vi "Mod_OFDM_Set_Ofdm_Frame.vi"(0 "Configure Variant":variant, 7 "ADD Symbol":T2, 9 "Add/delete":bool, 11 "error in":errorcluster, 12 "Edit Position":cluster{"Row":i32, "Column":i32}={"Row"=1000, "Column"=0} {"Row" min=0}) -> (4 "Configure Variant":variant, 8 "OFDM Frame":T1(array[cluster]), 15 "error out":errorcluster)   [LabVIEW 2010]
uses:
  Controls(Type_DEf)/Attribute Data Types.ctl
  Controls(Type_DEf)/Configure Pulse Shaping.ctl
  Controls(Type_DEf)/Pool of Modulator Control.ctl
  Controls(Type_DEf)/Pool of Data Source Control.ctl
  Controls(Type_DEf)/Attribute Names.ctl
  Mod_OFDM_Get_OFDM_Frame.vi
panel:
  in  "Attribute Data Types":T3={"Pulse Shaping"={"System Filter"={"TX Filter"=enum."none", "Alpha"=0.0, "filter length"=0}, "Modulation system parameters"={"samples per symbol (16)"=0}, "symbol rate (Hz)"=0.0}, "FRAME Table"=[], "OFDM Frame"=[], "Sub Carrier Selection"={"Sub Carrier Selection"=[], "OFDM Parameters"={"# of Sub Carrier"=0, "Length Of Cylic Prefix"=0}}, "Symbol Table"=[], "Symbol Pool"=[], "Pool of Modulators"=[], "Pool of Data Sources"=[], "Atribute Names"={"Data Source Pool"="Data Source Pool ", "Modulator Source Pool"="Modulator Source Pool ", "OFDM SYMBOL POOL"="OFDM SYMBOL POOL", "Symbol Table"="Symbol Table", "Sub Carrier Selection"="Sub Carrier Selection", "OFDM Frame"="OFDM Frame", "FRAME Table"="FRAME Table", "Pulse Shaping"="Pulse Shaping"}} {"Pool of Data Sources"."Register Initial State" format="%08x"; "Pulse Shaping"."symbol rate (Hz)" min=1.0 step=1.0 format="%.2p"; "Pulse Shaping"."Modulation system parameters"."samples per symbol (16)" step=2; "Pulse Shaping"."System Filter"."Alpha" min=0.0 max=1.0 step=0.05 format="%.2f"}
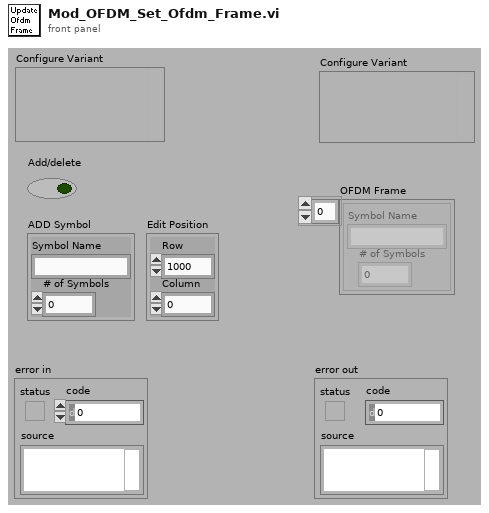
[diagram p1: front panel]
types:
  T1 = cluster{"Symbol Name":string, "# of Symbols":i32}[]
  T2 = cluster{"Symbol Name":string, "# of Symbols":i32}
  T3 = typedef "Attribute Data Types.ctl" = cluster{"Pulse Shaping":T4, "FRAME Table":string[][], "OFDM Frame":cluster{"Symbol Name":string, "# of Symbols":i32}[], "Sub Carrier Selection":cluster{"Sub Carrier Selection":cluster{"Sub Carrier":bool, "Data Source":u16, "Modulator":u16}[], "OFDM Parameters":cluster{"# of Sub Carrier":i32, "Length Of Cylic Prefix":i32}}, "Symbol Table":string[][], "Symbol Pool":string[], "Pool of Modulators":T5, "Pool of Data Sources":T6, "Atribute Names":T7}
  T4 = typedef "Configure Pulse Shaping.ctl" = cluster{"System Filter":cluster{"TX Filter":enum16{"none", "Raised Cosine", "Root Raised Cos"}, "Alpha":dbl, "filter length":i32}, "Modulation system parameters":cluster{"samples per symbol (16)":u32}, "symbol rate (Hz)":dbl}
  T5 = typedef "Pool of Modulator Control.ctl" = cluster{"M-QAM":enum16{"4", "16", "64", "256"}, "M-PSK":enum16{"2", "4", "8", "16", "32", "64", "128", "256"}, "Type of Modulation":enum16{"PSK", "QAM"}, " PSK":cluster{"differential PSK":enum16{"disable", "enable"}, "PSK type":enum16{"normal", "shifted", "offset"}}}[]
  T6 = typedef "Pool of Data Source Control.ctl" = cluster{"mode (PN)":enum16{"PN", "pattern", "user"}, "PN sequence order (9)":i32, "Invert Output Bits":enum16{"No", "Yes"}, "Register Initial State ":u32, "User base bit pattern":i8[], "base bit pattern (00001111)":enum16{"0", "1", "01", "0011", "00001111"}, "Reset to Initial State":enum16{"Every OFDM Frame", "Every OFDM Symbol", "Every Sub Carrier"}}[]
  T7 = typedef "Attribute Names.ctl" = cluster{"Data Source Pool":string, "Modulator Source Pool":string, "OFDM SYMBOL POOL":string, "Symbol Table":string, "Sub Carrier Selection":string, "OFDM Frame":string, "FRAME Table":string, "Pulse Shaping":string}
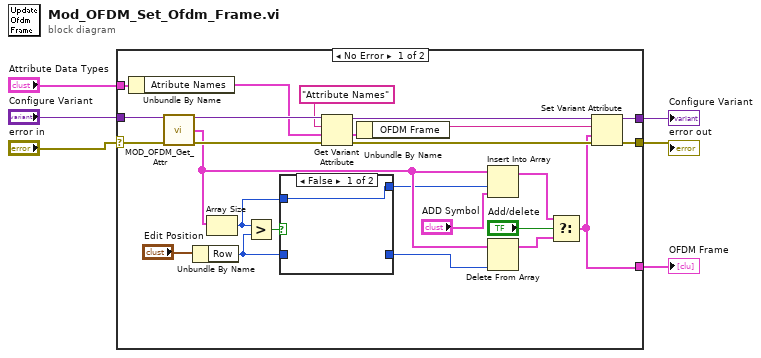
[diagram p0: block diagram]
diagram:
  n1 = case shown="No Error" "error in" {
    selector: "error in" -> [w27 w34]
    tunnel: "Configure Variant" -> [w31 _]
    tunnel: [w16 w34] -> w5
    tunnel: [w17 _] -> w4
    tunnel: "Attribute Data Types" -> [w26 _]
    tunnel: [w15 _] -> w1
    frame No Error {
      n2 = Unbundle By Name(w26) -> ("Atribute Names"=w21:T7)
      n3 = call-poly "MOD_OFDM_Get_Attr.vi"("Configuration in"=w31, "error in"=w27) -> ("Configuration out"=w24:variant, "OFDM Frame"=w12:T1, "error out"=w25:errorcluster)  [unwired: 10 in, 1 out]
      n4 = Unbundle By Name("Edit Position") -> ("Row"=w10:i32)
      n5 = Array Size(array=w12) -> (size(s)=w9:i32)
      n6 = Greater?(x=w9, y=w10) -> (0:w11:bool)
      n7 = case shown="False" w11 {
        tunnel: w10 -> [_ w33]
        tunnel: w9 -> [w32 _]
        tunnel: [_ w33] -> w8
        tunnel: [w32 w33] -> w7
        frame False {
        }
        frame True {
        }
      }
      n8 = Get Variant Attribute(Variant=w24, name="Attribute Names", default value (empty Variant)=w21, error in=w25) -> (duplicate Variant=w23:variant, value=w19:T7, error out=w22:errorcluster)  [unwired: 1 out]
      n9 = Unbundle By Name(w19) -> ("OFDM Frame"=w18:string)
      n10 = Insert Into Array(array=w12, index=w7, new element="ADD Symbol") -> (w29:T1)
      n11 = Delete From Array(array=w12, index=w8) -> (array with subset deleted=w28:T1)  [unwired: 1 in, 1 out]
      n12 = Select(t=w29, s="Add/delete", f=w28) -> (s? t:f=w15:T1)
      n13 = Set Variant Attribute(Variant=w23, name=w18, value=w15, error in=w22) -> (Variant out=w17:variant, error out=w16:errorcluster)  [unwired: 1 out]
    }
    frame Error {
    }
  }
  "Configure Variant" <- w4
  "error out" <- w5
  "OFDM Frame" <- w1
